vi "LB_GetRGBI.vi"(8 "error in (no error)":errorcluster caption="错误输入（无错误）", 10 "CH":u8=1 min=1, 11 "LB_COM_IN":refnum<visa-resource-name>="COM4") -> (0 "error out":errorcluster caption="错误输出", 1 "Blue":u8, 2 "Green":u8, 3 "LB_COM_OUT":refnum<visa-resource-name>, 4 "Lightness":u32, 5 "Red":u8, 7 "OK":bool)   [LabVIEW 2015, in "LBAnalyser.lvlib"]
uses:
  LBAnalyser.lvlib
  UartCOM/UARTCOM.lvlib
panel:
  out "Color":u32(colorbox) caption="颜色"
  out "读取字符串":string
  # ">=1"
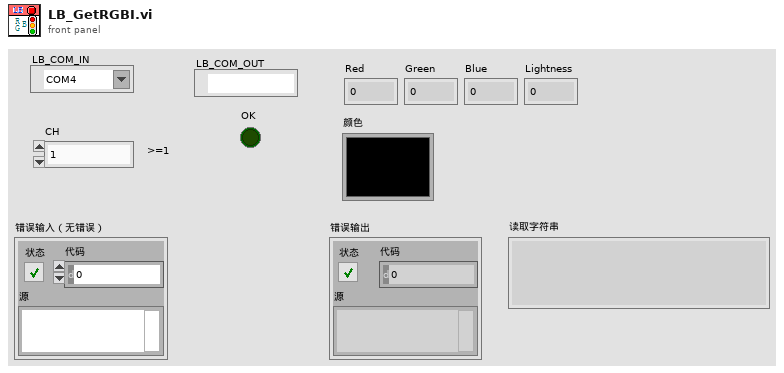
[diagram p1: front panel]
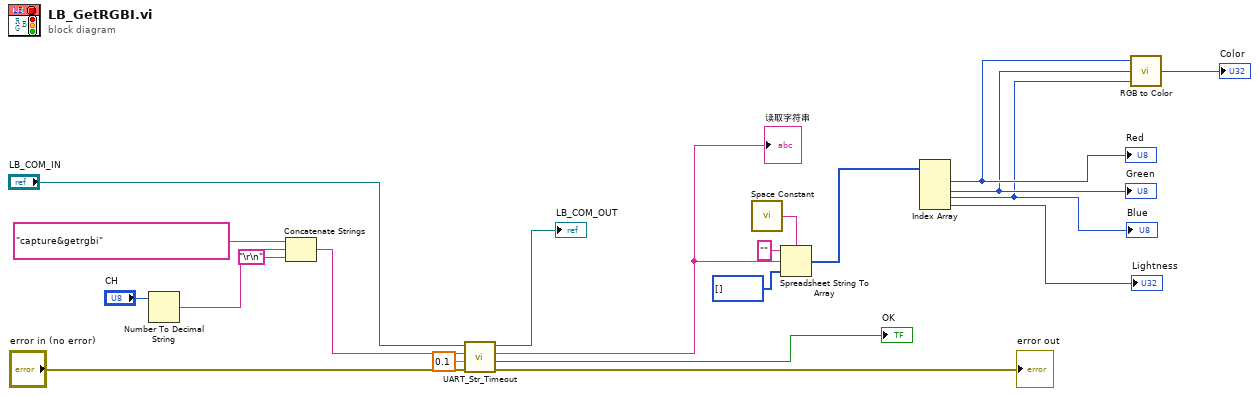
[diagram p0: block diagram]
diagram:
  n1 = Number To Decimal String(number="CH") -> (decimal integer string=w17:string)  [unwired: 1 in]
  n2 = Concatenate Strings("capture&getrgbi" ("写入字符串"), w17, "\r\n") -> (w15:string)
  n3 = call "UART_Str_Timeout.vi"("error in (no error)"="error in (no error)", "超时s"=0.1, "写入字符串"=w15, "BASE_COM"="LB_COM_IN") -> ("error out"=→"error out":errorcluster, "OK"=→"OK":bool, "读取字符串"=w13:string, "BASE_COM_OUT"=→"LB_COM_OUT":refnum<visa-resource-name>)  [unwired: 3 in, 1 out]
  "读取字符串" <- w13
  n4 = call <vilib>:"Space Constant.vi"() -> ("String"=w11:string)
  n5 = Spreadsheet String To Array(delimiter (Tab)=w11, format string="" ("格式字符串"), spreadsheet string=w13, array type (2D Dbl)=u32[] []) -> (array=w7:u32[])
  n6 = Index Array(array=w7) -> (element #1=w5:u32, element #2=w4:u32, element #3=w3:u32, element #4=→"Lightness":u32)  [unwired: 4 in]
  "Red" <- w5
  "Green" <- w4
  "Blue" <- w3
  n7 = call <vilib>:"RGB to Color.vi"("B"=w3, "G"=w4, "R"=w5) -> ("Color"=→"Color":u32)
